vi "TemperatureReadout.vi"(0 "Handle In":i32, 1 "TC1 +Channel":u16, 2 "TC1 -Channel":u16, 5 "TC1 Type":u16(ring) items=["B", "E", "J", "K", "N", "R", "S", "T"], 9 "TC2 Type":u16(ring) items=["B", "E", "J", "K", "N", "R", "S", "T"], 11 "error in":errorcluster, 12 "TC2 +Channel":u16, 13 "TC2 -Channel":u16) -> (3 "TC1 Raw Readings":dbl format="%.6f", 4 "TC1 Temperature (Deg F)":dbl format="%.2f", 6 "TC1 Temperature (Deg C)":dbl format="%.2f", 8 "TC2 Temperature (Deg C)":dbl format="%.2f", 10 "TC2 Temperature (Deg F)":dbl format="%.2f", 14 "TC2 Raw Readings":dbl format="%.6f", 15 "error out":errorcluster[](array[cluster]))   [LabVIEW 2021]
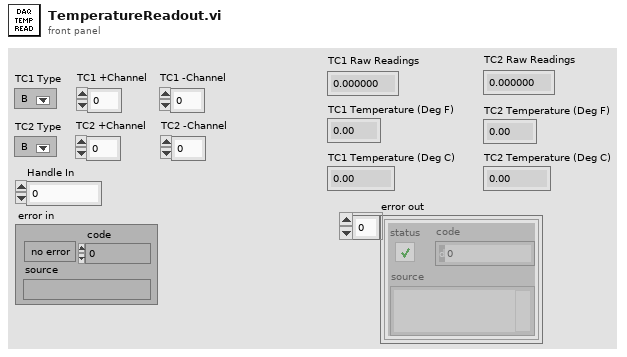
[diagram p1: front panel]
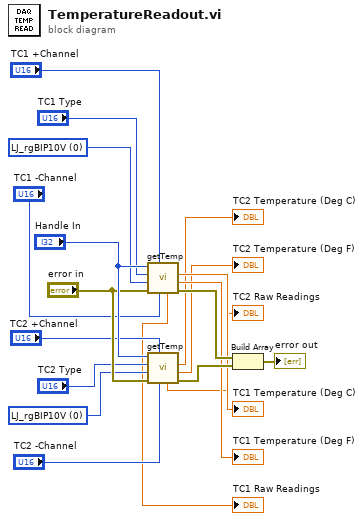
[diagram p0: block diagram]
diagram:
  w16 = u16 0 items=["LJ_rgBIP10V", "LJ_rgBIP1V", "LJ_rgBIPP1V", "LJ_rgBIPP01V"] ("AIN Range")
  w17 = u16 0 items=["LJ_rgBIP10V", "LJ_rgBIP1V", "LJ_rgBIPP1V", "LJ_rgBIPP01V"] ("AIN Range")
  n1 = call "getTemp.vi"("-Channel"="TC1 -Channel", "+Channel"="TC1 +Channel", "error in"="error in", "AIN Range"=w17, "Thermocouple Type"="TC1 Type", "Handle In"="Handle In") -> ("error out"=w9:errorcluster, "Temperature (Deg F)"=→"TC1 Temperature (Deg F)":dbl, "Temperature (Deg C)"=→"TC1 Temperature (Deg C)":dbl, "Raw Readings"=→"TC1 Raw Readings":dbl)  [unwired: 1 in, 1 out]
  n2 = call "getTemp.vi"("-Channel"="TC2 -Channel", "+Channel"="TC2 +Channel", "error in"="error in", "AIN Range"=w16, "Thermocouple Type"="TC2 Type", "Handle In"="Handle In") -> ("error out"=w8:errorcluster, "Temperature (Deg F)"=→"TC2 Temperature (Deg F)":dbl, "Temperature (Deg C)"=→"TC2 Temperature (Deg C)":dbl, "Raw Readings"=→"TC2 Raw Readings":dbl)  [unwired: 1 in, 1 out]
  n3 = Build Array(w9, w8) -> (→"error out":errorcluster[])
